vi "Set_up_waveform.vi"(5 "TimeOut Time (s)":dbl=30.0 format="%.2f", 7 "DataSocketCluster In":T1={"Server Machine"="siskin", "Client Machine"="becard", "Data"="P2", "TimeStamp"=0.0, "Count"=0, "Target Process"="General Server"} {"TimeStamp" format="%.2f"}, 8 "error in (no error)":errorcluster, 9 "Steps on PJVS curve":u32=100, 10 "Frequency (Hz)":dbl=100.0, 11 "Amplitude (V)":dbl=1.0) -> (0 "error IO":errorcluster, 1 "Returned number of steps on PJVS curve":string, 2 "Set frequency (Hz)":dbl=100.0, 3 "Voltage at each step on PJVS curve":dbl[](array[numeric]) format="%#_16g", 4 "Calculated time on step (smallest value is 17)":u32=100, 6 "Returned time interval on each step":string)   [LabVIEW 2020]
uses:
  DataSocketCluster external.ctl
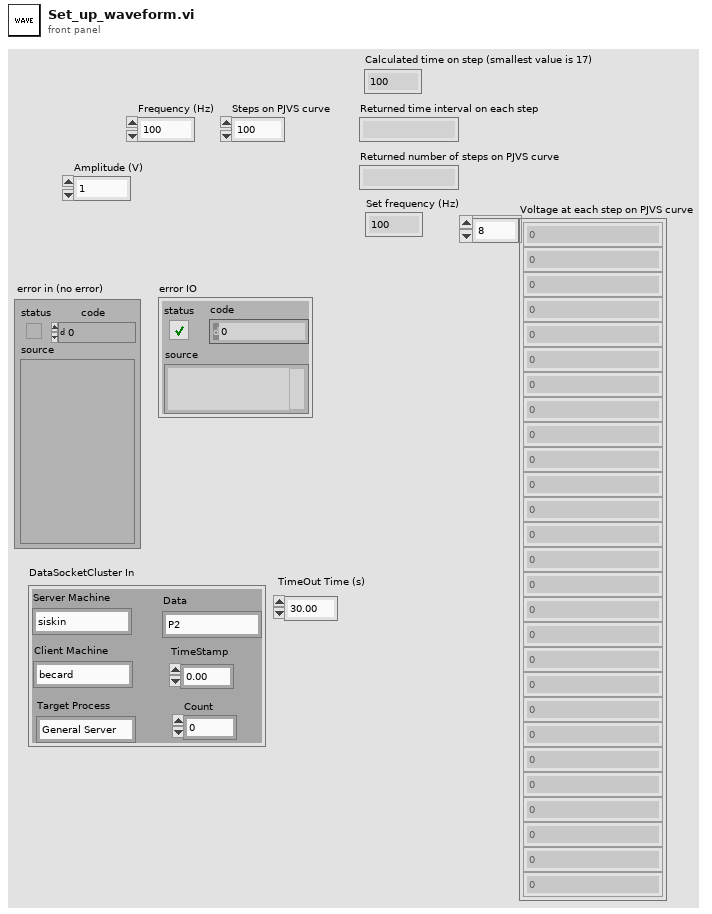
[diagram p1: front panel]
types:
  T1 = typedef "DataSocketCluster external.ctl" = cluster{"Server Machine":string, "Client Machine":string, "Data":string, "TimeStamp":dbl, "Count":i32, "Target Process":string}
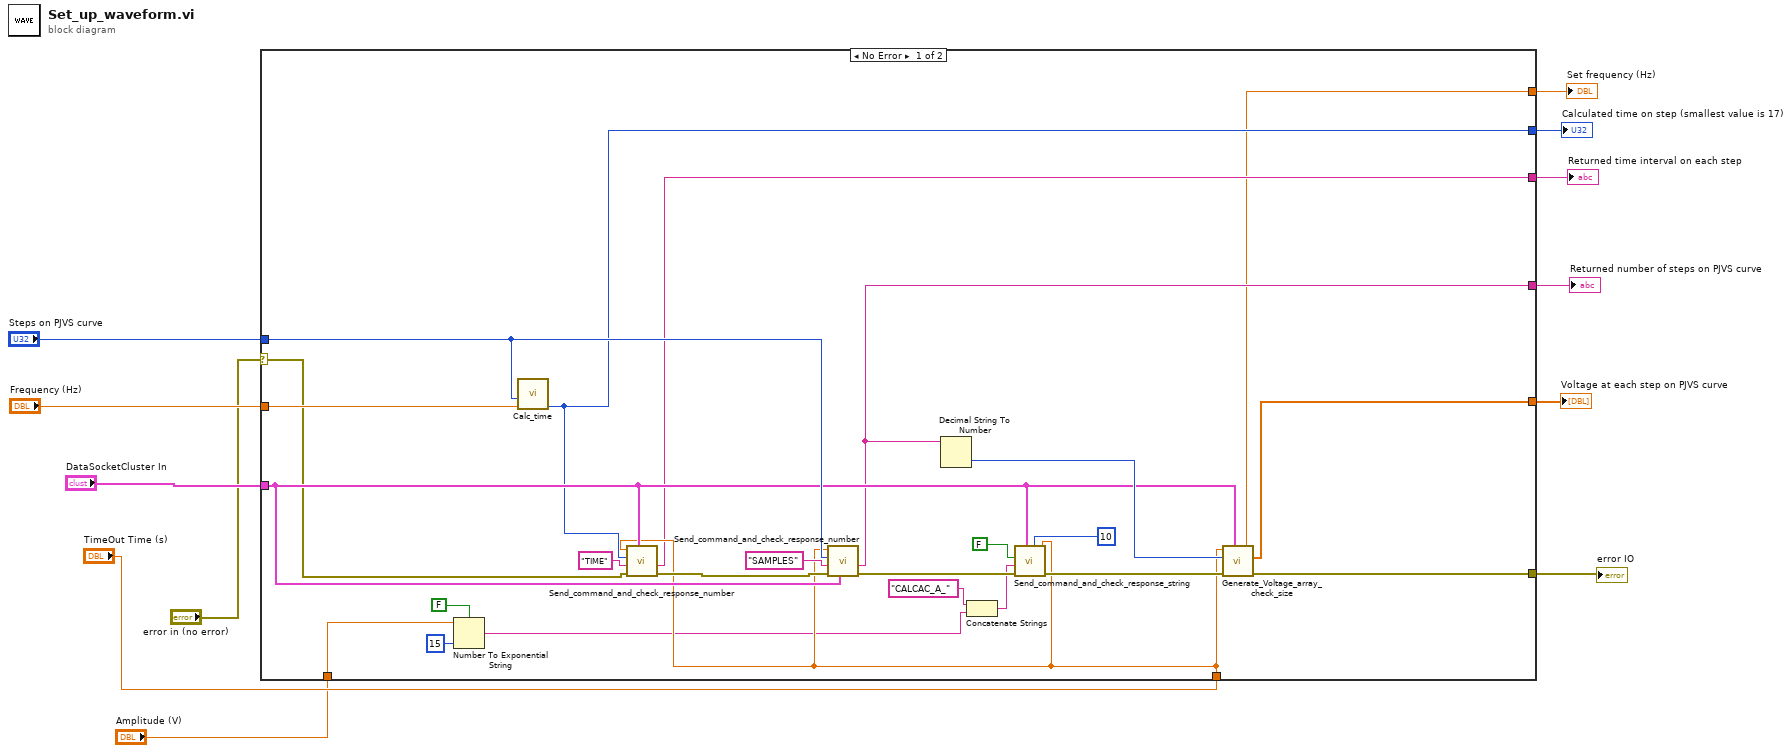
[diagram p0: block diagram]
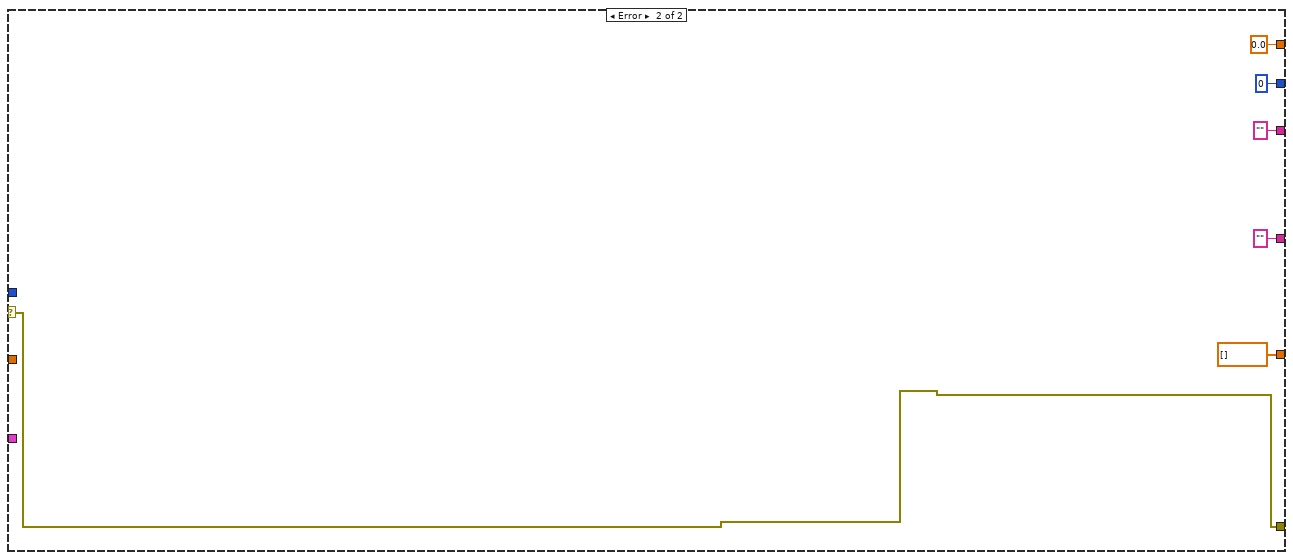
[diagram p2: hidden frame]
diagram:
  n1 = case shown="No Error" "error in (no error)" {
    selector: "error in (no error)" -> [w17 w38]
    tunnel: "Steps on PJVS curve" -> [w31 _]
    tunnel: [w26 w38] -> w12
    tunnel: "DataSocketCluster In" -> [w25 _]
    tunnel: "TimeOut Time (s)" -> [w24 _]
    tunnel: "Frequency (Hz)" -> [w23 _]
    tunnel: [w22 dbl[] [] ("Voltage at each step on PJVS curve 2")] -> w8
    tunnel: [w21 "" ("Return value")] -> w7
    tunnel: [w20 "" ("Return value")] -> w6
    tunnel: [w19 0 ("Time")] -> w5
    tunnel: [w18 0.0 ("Frequency Out (Hz)")] -> w4
    tunnel: "Amplitude (V)" -> [w14 _]
    frame No Error {
      n2 = Number To Exponential String(number=w14, precision (6)=i16 15, 1:FALSE ("use system decimal point (T)")) -> (E-format string=w13:string)  [unwired: 1 in]
      n3 = call "Calc_time.vi"("Frequency"=w23, "Steps on PJVS curve"=w31) -> ("Time"=w19:i32)  [unwired: 8 in, 1 out]
      n4 = call "Send_command_and_check_response_number.vi"("output cluster"=w25, "error in (no error)"=w17, "Command"="TIME", "Set value"=w19, "TimeOut Time (s)"=w24) -> ("error IO"=w34:errorcluster, "Return value"=w20:string)  [unwired: 3 in]
      n5 = call "Send_command_and_check_response_number.vi"("output cluster"=w25, "error in (no error)"=w34, "Command"="SAMPLES", "Set value"=w31, "TimeOut Time (s)"=w24) -> ("error IO"=w35:errorcluster, "Return value"=w21:string)  [unwired: 3 in]
      n6 = Decimal String To Number(string=w21) -> (number=w27:i32)  [unwired: 2 in, 1 out]
      n7 = Concatenate Strings("CALCAC_A_", w13) -> (w30:string)
      n8 = call "Send_command_and_check_response_string.vi"("TimeOut Time (s)"=w24, "milliseconds to wait"=u32 10, "output cluster"=w25, "error in (no error)"=w35, "Command"=w30, "test response?"=FALSE) -> ("error IO"=w36:errorcluster)  [unwired: 2 in, 1 out]
      n9 = call "Generate_Voltage_array_check_size.vi"("output cluster"=w25, "error in (no error)"=w36, "Number of Steps"=w27, "TimeOut Time (s)"=w24) -> ("error IO"=w26:errorcluster, "Voltage at each step on PJVS curve 2"=w22:dbl[], "Set Frequency"=w18:dbl)  [unwired: 1 in, 1 out]
    }
    frame Error {
    }
  }
  "error IO" <- w12
  "Voltage at each step on PJVS curve" <- w8
  "Returned number of steps on PJVS curve" <- w7
  "Returned time interval on each step" <- w6
  "Calculated time on step (smallest value is 17)" <- w5
  "Set frequency (Hz)" <- w4
